vi "MecaDrivePoseEst_Update.vi"(6 "MecanumWheelPositions":T1 {"RearRight" format="%19.3f"; "RearLeft" format="%19.3f"; "FrontRight" format="%19.3f"; "FrontLeft" format="%19.3f"}, 8 "MecanumWheelSpeeds":T2 {"RearRightSpeed" format="%19.3f"; "RearLeftSpeed" format="%19.3f"; "FrontRightSpeed" format="%19.3f"; "FrontLeftSpeed" format="%19.3f"}, 9 "GyroAngle":T5={"VALUE"=0.0, "COS"=1.0, "SIN"=0.0} {"SIN" format="%13.4f"; "COS" format="%13.4f"; "VALUE" format="%13.4f"}, 10 "Time":dbl=-1.0 format="%33.4f", 11 "in MecaDrivePoseEstimate":T6={"M_VisionContR"=[], "m_nominal_dT"=0.0, "m_PrevTime_Sec"=0.0, "m_GyroOffset"={"VALUE"=0.0, "COS"=1.0, "SIN"=0.0}, "m_PrevAngle"={"VALUE"=0.0, "COS"=1.0, "SIN"=0.0}, "m_Observer"={"m_P"=[], "m_xHat"=[], "States"=0, "Outputs"=0, "m_ContR"=[], "m_ContQ"=[], "m_SigmasF"=[], "m_dT_Sec"=0.0, "MERWE_SCALED_SIGMA_PTS"={"m_Wm"=[], "States"=0, "Alpha"=0.0, "m_Wc"=[], "Kappa"=0}, "meanFuncX"=refnum, "meanFuncY"=refnum, "residualFuncX"=refnum, "residualFuncY"=refnum, "addFuncX"=refnum, "addFuncXExtra"=variant, "residualFuncYExtra"=variant, "residualFuncXExtra"=variant, "MeanFuncYExtra"=variant, "MeanFuncXExtra"=variant, "Inputs"=0}, "m_kinematics"={"FrontLeft"={"X"=0.0, "Y"=0.0}, "FrontRight"={"X"=0.0, "Y"=0.0}, "RearLeft"={"X"=0.0, "Y"=0.0}, "RearRight"={"X"=0.0, "Y"=0.0}, "InverseKinematics"=[[0.0, 1.0, -1.0, 0.0], [0.0, 1.0, 1.0, 0.0], [0.0, 1.0, 1.0, 0.0], [0.0, 1.0, -1.0, 0.0]], "ForwardKinematics"=[[0.0, 1.0, -1.0, 0.0], [0.0, 1.0, 1.0, 0.0], [0.0, 1.0, 1.0, 0.0], [0.0, 1.0, -1.0, 0.0]], "PrevCoR"={"X"=0.0, "Y"=0.0}}, "Pose_Buffer"={"TimeStamps"=[], "Pose"=[], "Min_TimeStamp"=0.0, "Max_TimeStamp"=0.0, "ItemCount"=0, "MaxBufferTime"=0.0}} {"Pose_Buffer"."Pose"."ROTATION"."SIN" format="%13.4f"; "Pose_Buffer"."Pose"."ROTATION"."COS" format="%13.4f"; "Pose_Buffer"."Pose"."ROTATION"."VALUE" format="%13.4f"; "Pose_Buffer"."Pose"."TRANSLATION"."Y" format="%14.3f"; "Pose_Buffer"."Pose"."TRANSLATION"."X" format="%14.3f"; "m_kinematics"."PrevCoR"."Y" format="%14.3f"; "m_kinematics"."PrevCoR"."X" format="%14.3f"; "m_kinematics"."RearRight"."Y" format="%14.3f"; "m_kinematics"."RearRight"."X" format="%14.3f"; "m_kinematics"."RearLeft"."Y" format="%14.3f"; "m_kinematics"."RearLeft"."X" format="%14.3f"; "m_kinematics"."FrontRight"."Y" format="%14.3f"; "m_kinematics"."FrontRight"."X" format="%14.3f"; "m_kinematics"."FrontLeft"."Y" format="%14.3f"; "m_kinematics"."FrontLeft"."X" format="%14.3f"; "m_PrevAngle"."SIN" format="%13.4f"; "m_PrevAngle"."COS" format="%13.4f"; "m_PrevAngle"."VALUE" format="%13.4f"; "m_GyroOffset"."SIN" format="%13.4f"; "m_GyroOffset"."COS" format="%13.4f"; "m_GyroOffset"."VALUE" format="%13.4f"}) -> (0 "Error":bool, 2 "Estimated Pose":T3 {"ROTATION"."SIN" format="%13.4f"; "ROTATION"."COS" format="%13.4f"; "ROTATION"."VALUE" format="%13.4f"; "TRANSLATION"."Y" format="%14.3f"; "TRANSLATION"."X" format="%14.3f"}, 3 "Out MecaDrivePoseEstimate":T6={"M_VisionContR"=[], "m_nominal_dT"=0.0, "m_PrevTime_Sec"=0.0, "m_GyroOffset"={"VALUE"=0.0, "COS"=1.0, "SIN"=0.0}, "m_PrevAngle"={"VALUE"=0.0, "COS"=1.0, "SIN"=0.0}, "m_Observer"={"m_P"=[], "m_xHat"=[], "States"=0, "Outputs"=0, "m_ContR"=[], "m_ContQ"=[], "m_SigmasF"=[], "m_dT_Sec"=0.0, "MERWE_SCALED_SIGMA_PTS"={"m_Wm"=[], "States"=0, "Alpha"=0.0, "m_Wc"=[], "Kappa"=0}, "meanFuncX"=refnum, "meanFuncY"=refnum, "residualFuncX"=refnum, "residualFuncY"=refnum, "addFuncX"=refnum, "addFuncXExtra"=variant, "residualFuncYExtra"=variant, "residualFuncXExtra"=variant, "MeanFuncYExtra"=variant, "MeanFuncXExtra"=variant, "Inputs"=0}, "m_kinematics"={"FrontLeft"={"X"=0.0, "Y"=0.0}, "FrontRight"={"X"=0.0, "Y"=0.0}, "RearLeft"={"X"=0.0, "Y"=0.0}, "RearRight"={"X"=0.0, "Y"=0.0}, "InverseKinematics"=[[0.0, 1.0, -1.0, 0.0], [0.0, 1.0, 1.0, 0.0], [0.0, 1.0, 1.0, 0.0], [0.0, 1.0, -1.0, 0.0]], "ForwardKinematics"=[[0.0, 1.0, -1.0, 0.0], [0.0, 1.0, 1.0, 0.0], [0.0, 1.0, 1.0, 0.0], [0.0, 1.0, -1.0, 0.0]], "PrevCoR"={"X"=0.0, "Y"=0.0}}, "Pose_Buffer"={"TimeStamps"=[], "Pose"=[], "Min_TimeStamp"=0.0, "Max_TimeStamp"=0.0, "ItemCount"=0, "MaxBufferTime"=0.0}} {"Pose_Buffer"."Pose"."ROTATION"."SIN" format="%13.4f"; "Pose_Buffer"."Pose"."ROTATION"."COS" format="%13.4f"; "Pose_Buffer"."Pose"."ROTATION"."VALUE" format="%13.4f"; "Pose_Buffer"."Pose"."TRANSLATION"."Y" format="%14.3f"; "Pose_Buffer"."Pose"."TRANSLATION"."X" format="%14.3f"; "m_kinematics"."PrevCoR"."Y" format="%14.3f"; "m_kinematics"."PrevCoR"."X" format="%14.3f"; "m_kinematics"."RearRight"."Y" format="%14.3f"; "m_kinematics"."RearRight"."X" format="%14.3f"; "m_kinematics"."RearLeft"."Y" format="%14.3f"; "m_kinematics"."RearLeft"."X" format="%14.3f"; "m_kinematics"."FrontRight"."Y" format="%14.3f"; "m_kinematics"."FrontRight"."X" format="%14.3f"; "m_kinematics"."FrontLeft"."Y" format="%14.3f"; "m_kinematics"."FrontLeft"."X" format="%14.3f"; "m_PrevAngle"."SIN" format="%13.4f"; "m_PrevAngle"."COS" format="%13.4f"; "m_PrevAngle"."VALUE" format="%13.4f"; "m_GyroOffset"."SIN" format="%13.4f"; "m_GyroOffset"."COS" format="%13.4f"; "m_GyroOffset"."VALUE" format="%13.4f"})   [LabVIEW 2019, in "Trajectory_Library.lvlib"]
doc: "Updates the the Unscented Kalman Filter using only wheel encoder information. This should be called every loop, and the correct loop period must be passed into the constructor of this class.\n\nInputs:\n - In Meca Pose Est -- Input data cluster. \n - gyroAngle -- The current gyro angle.\n - wheelSpeeds -- The current velocities wheels.\n - wheelPositions -- The distances driven by each wheel.\n - currentTimeSeconds -- (Optional) Time at which this method was called, in seconds.\n\nOutputs:\n - outMecaPoseEst -- Updated data cluster \n - EstimatedPose -- The estimated pose of the robot in meters.\n - Error -- If TRUE, an error occured."
uses:
  Trajectory_Library.lvlib
  <vilib>/Analysis/Matrix/Datatypes/RealMatrix.ctl
  <vilib>/Analysis/Matrix/NI_Matrix.lvlib
  TypeDef/MERWE_SCALED_SIGMA_PTS.ctl
  TypeDef/UNSCENTED_KALMAN_FILTER.ctl
  TypeDef/CALLBACK_FUNC_TYPE.ctl
  TypeDef/ROTATION2D.ctl
  TypeDef/TRANSLATION2D.ctl
  TypeDef/POSE2D.ctl
  TypeDef/TIME_INTERPOLATABLE_POSE2D.ctl
  TypeDef/MECA_DRIVE_KINEMATICS.ctl
  TypeDef/MECA_DRIVE_POSE_EST.ctl
  TypeDef/MECA_WHEEL_SPEEDS.ctl
  TypeDef/MECA_WHEEL_POSITIONS.ctl
panel:
  # "<3, 3>"
  # "State Estimate <Statess,1>"
  # "<States, States>"
  # "<States, ?>"
  # "<Statess,  States>"
  # "<Outputs, Outputs>"
  # "<?, 1>"
  # "<?, 1>"
  # "<3, 3>"
  # "State Estimate <Statess,1>"
  # "<States, States>"
  # "<States, ?>"
  # "<Statess,  States>"
  # "<Outputs, Outputs>"
  # "<?, 1>"
  # "<?, 1>"
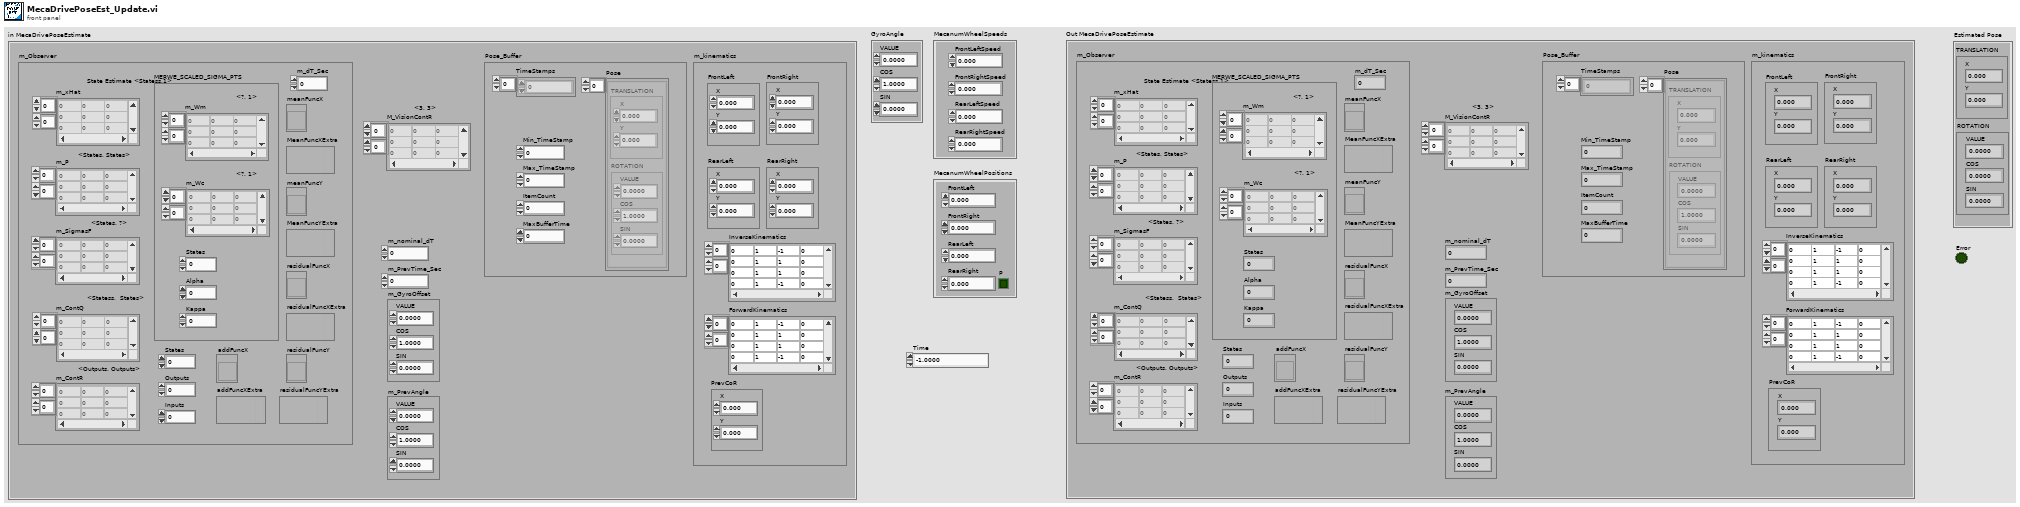
[diagram p1: front panel]
types:
  T1 = typedef "Trajectory_Library.lvlib/MECA_WHEEL_POSITIONS.ctl" = cluster{"FrontLeft":dbl, "FrontRight":dbl, "RearLeft":dbl, "RearRight":dbl, "P":bool}
  T2 = typedef "Trajectory_Library.lvlib/MECA_WHEEL_SPEEDS.ctl" = cluster{"FrontLeftSpeed":dbl, "FrontRightSpeed":dbl, "RearLeftSpeed":dbl, "RearRightSpeed":dbl}
  T3 = typedef "Trajectory_Library.lvlib/POSE2D.ctl" = cluster{"TRANSLATION":T4, "ROTATION":T5}
  T4 = typedef "Trajectory_Library.lvlib/TRANSLATION2D.ctl" = cluster{"X":dbl, "Y":dbl}
  T5 = typedef "Trajectory_Library.lvlib/ROTATION2D.ctl" = cluster{"VALUE":dbl, "COS":dbl, "SIN":dbl}
  T6 = typedef "Trajectory_Library.lvlib/MECA_DRIVE_POSE_EST.ctl" = cluster{"M_VisionContR":T7, "m_nominal_dT":dbl, "m_PrevTime_Sec":dbl, "m_GyroOffset":T5, "m_PrevAngle":T5, "m_Observer":T8, "m_kinematics":T11, "Pose_Buffer":T12}
  T7 = typedef "NI_Matrix.lvlib/RealMatrix.ctl" = dbl[][]
  T8 = typedef "Trajectory_Library.lvlib/UNSCENTED_KALMAN_FILTER.ctl" = cluster{"m_P":T7, "m_xHat":T7, "States":i32, "Outputs":i32, "m_ContR":T7, "m_ContQ":T7, "m_SigmasF":T7, "m_dT_Sec":dbl, "MERWE_SCALED_SIGMA_PTS":T9, "meanFuncX":T10, "meanFuncY":T10, "residualFuncX":T10, "residualFuncY":T10, "addFuncX":T10, "addFuncXExtra":variant, "residualFuncYExtra":variant, "residualFuncXExtra":variant, "MeanFuncYExtra":variant, "MeanFuncXExtra":variant, "Inputs":i32}
  T9 = typedef "Trajectory_Library.lvlib/MERWE_SCALED_SIGMA_PTS.ctl" = cluster{"m_Wm":T7, "States":i32, "Alpha":dbl, "m_Wc":T7, "Kappa":i32}
  T10 = typedef "Trajectory_Library.lvlib/CALLBACK_FUNC_TYPE.ctl" = refnum<vi>
  T11 = typedef "Trajectory_Library.lvlib/MECA_DRIVE_KINEMATICS.ctl" = cluster{"FrontLeft":T4, "FrontRight":T4, "RearLeft":T4, "RearRight":T4, "InverseKinematics":T7, "ForwardKinematics":T7, "PrevCoR":T4}
  T12 = typedef "Trajectory_Library.lvlib/TIME_INTERPOLATABLE_POSE2D.ctl" = cluster{"TimeStamps":dbl[], "Pose":T3[], "Min_TimeStamp":dbl, "Max_TimeStamp":dbl, "ItemCount":i32, "MaxBufferTime":dbl}
  T13 = typedef "WPILib_Math.lvlib/POSE2D.ctl" = cluster{"TRANSLATION":T14, "ROTATION":T15}
  T14 = typedef "WPILib_Math.lvlib/TRANSLATION2D.ctl" = cluster{"X":dbl, "Y":dbl}
  T15 = typedef "WPILib_Math.lvlib/ROTATION2D.ctl" = cluster{"VALUE":dbl, "COS":dbl, "SIN":dbl}
  T16 = typedef "WPILib_Math.lvlib/MECA_DRIVE_POSE_EST.ctl" = cluster{"M_VisionContR":T7, "m_nominal_dT":dbl, "m_PrevTime_Sec":dbl, "m_GyroOffset":T15, "m_PrevAngle":T15, "m_Observer":T17, "m_kinematics":T20, "Pose_Buffer":T21}
  T17 = typedef "WPILib_Math.lvlib/UNSCENTED_KALMAN_FILTER.ctl" = cluster{"m_P":T7, "m_xHat":T7, "States":i32, "Outputs":i32, "m_ContR":T7, "m_ContQ":T7, "m_SigmasF":T7, "m_dT_Sec":dbl, "MERWE_SCALED_SIGMA_PTS":T18, "meanFuncX":T19, "meanFuncY":T19, "residualFuncX":T19, "residualFuncY":T19, "addFuncX":T19, "addFuncXExtra":variant, "residualFuncYExtra":variant, "residualFuncXExtra":variant, "MeanFuncYExtra":variant, "MeanFuncXExtra":variant, "Inputs":i32}
  T18 = typedef "WPILib_Math.lvlib/MERWE_SCALED_SIGMA_PTS.ctl" = cluster{"m_Wm":T7, "States":i32, "Alpha":dbl, "m_Wc":T7, "Kappa":i32}
  T19 = typedef "WPILib_Math.lvlib/CALLBACK_FUNC_TYPE.ctl" = refnum<vi>
  T20 = typedef "WPILib_Math.lvlib/MECA_DRIVE_KINEMATICS.ctl" = cluster{"FrontLeft":T14, "FrontRight":T14, "RearLeft":T14, "RearRight":T14, "InverseKinematics":T7, "ForwardKinematics":T7, "PrevCoR":T14}
  T21 = typedef "WPILib_Math.lvlib/TIME_INTERPOLATABLE_POSE2D.ctl" = cluster{"TimeStamps":dbl[], "Pose":T13[], "Min_TimeStamp":dbl, "Max_TimeStamp":dbl, "ItemCount":i32, "MaxBufferTime":dbl}
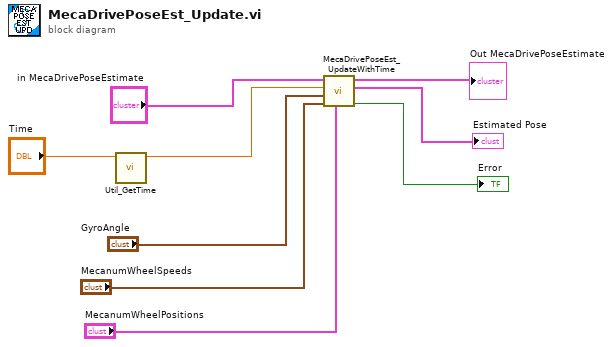
[diagram p0: block diagram]
diagram:
  n1 = call "Util_GetTime.vi"("Pass_Through_Time"="Time") -> ("FPGA_Time_Seconds"=w4:dbl)  [unwired: 9 in, 1 out]
  n2 = call "MecaDrivePoseEst_UpdateWithTime.vi"("MecanumWheelPositions"="MecanumWheelPositions", "MecanumWheelSpeeds"="MecanumWheelSpeeds", "GyroAngle"="GyroAngle", "CurrentTimeSeconds"=w4, "in MecaDrivePoseEstimate"="in MecaDrivePoseEstimate") -> ("Error"=→"Error":bool, "Estimated Pose"=→"Estimated Pose":T13, "Out MecaDrivePoseEstimate"=→"Out MecaDrivePoseEstimate":T16)  [unwired: 4 in]
